vi "Test Log Critical Message.vi"(8 "error in (no error)":errorcluster, 11 "Test Case In":refnum<class "Logger Test.lvclass">) -> (0 "error out":errorcluster, 3 "Test Case Out":refnum<class "Logger Test.lvclass">)   [LabVIEW 2020, in "Logger Test.lvclass"]
uses:
  Logger Test.lvclass
  Logger Test.lvclass/Logger Test.ctl
  source/Framework Test Suite/Mock Log Handler/Mock Log Handler.lvclass
  source/Framework/Process/Process.lvclass
  source/Framework Test Suite/Mock Process/Mock Process.lvclass
  source/Framework/Logging/Logging.lvclass
  C:/Git/astemes-triarc-framework/source/Framework/Process/Process.lvclass
  C:/Git/astemes-triarc-framework/source/Framework/Base/Base.lvclass
  C:/Git/astemes-triarc-framework/source/Framework/Configuration File/Configuration File.lvclass
  C:/Git/astemes-triarc-framework/source/Framework/Configuration/Configuration.lvclass
  C:/Git/astemes-triarc-framework/source/Framework/Error Handler Interface/Error Handler Interface.lvclass
  C:/Git/astemes-triarc-framework/source/Framework/Logging/Logging.lvclass
  C:/Git/astemes-triarc-framework/source/Framework Test Suite/Mock Process/Mock Process.lvclass
  C:/Git/astemes-triarc-framework/source/Framework/Async Handler/Async Handler.lvclass
  C:/Git/astemes-triarc-framework/source/Framework/Helper Loop/Helper Loop.lvclass
  2651e2de-d45e-4850-8bc5-6c099aad78ff.vi
  C:/Git/astemes-triarc-framework/source/Framework Test Suite/Mock Log Handler/Mock Log Handler.lvclass
  5330ea77-6064-4515-90a2-c99ab62f2416.vi
  b0e1ba43-fbce-4c73-8e5c-724704fff6a6.vi
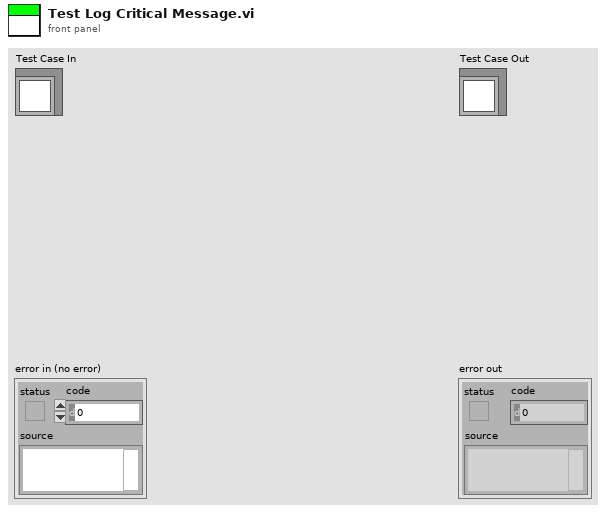
[diagram p1: front panel]
types:
  T1 = typedef "Mock Log Handler.lvclass/Log Entry.ctl" = cluster{"Level":string, "Source":string, "Message":string}
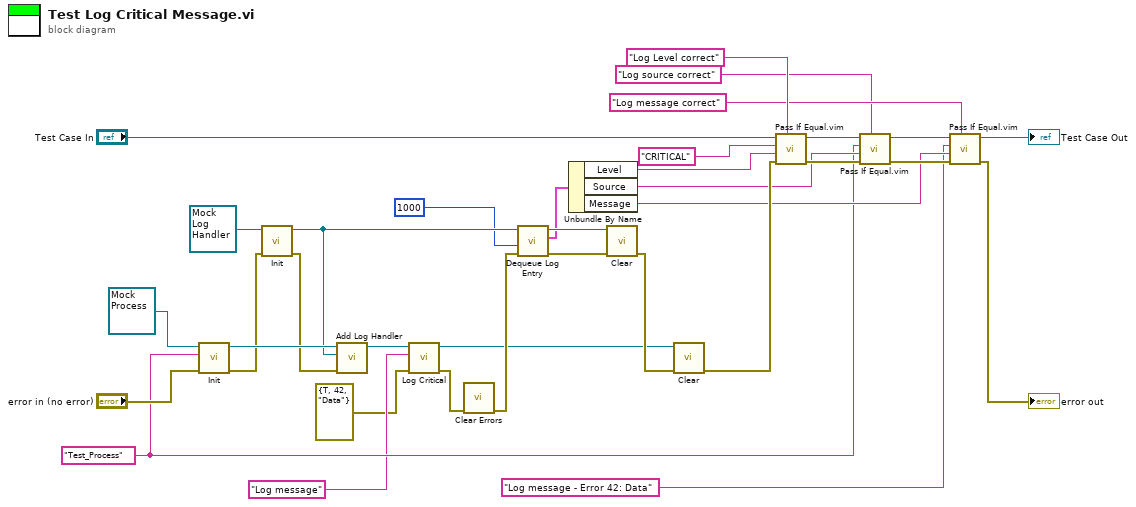
[diagram p0: block diagram]
diagram:
  w7 = "Test_Process" ("Name")
  n1 = call-dynamic "Init.vi"("error in (no error)"="error in (no error)", "Name"=w7, "Mock Process In"=refnum<class "Mock Process.lvclass"> refnum) -> ("error out"=w28:errorcluster, "Mock Process Out"=w32:refnum<class "Mock Process.lvclass">)  [unwired: 7 in]
  n2 = call-dynamic "Init.vi"("error in (no error)"=w28, "Mock Log Handler In"=refnum<class "Mock Log Handler.lvclass"> refnum ("Mock Log Handler.lvclass")) -> ("error out"=w27:errorcluster, "Mock Log Handler Out"=w24:refnum<class "Mock Log Handler.lvclass">)  [unwired: 8 in]
  n3 = call "Add Log Handler.vi"("error in (no error)"=w27, "Log Handler"=w24, "Process In"=w32) -> ("Process Out"=w22:refnum<class "Mock Process.lvclass">)  [unwired: 7 in, 1 out]
  n4 = call "Log Critical.vi"("error in (no error)"=errorcluster {"status"=TRUE, "code"=42, "source"="Data"}, "Message"="Log message", "Logging In"=w22) -> ("error out"=w4:errorcluster, "Logging Out"=w1:refnum<class "Mock Process.lvclass">)  [unwired: 7 in]
  n5 = call <vilib>:"Clear Errors.vi"("error in (no error)"=w4) -> ("error out"=w3:errorcluster)  [unwired: 5 in, 1 out]
  n6 = call "Dequeue Log Entry.vi"("error in (no error)"=w3, "timeout in ms (-1)"=1000, "Mock Log Handler in"=w24) -> ("error out"=w25:errorcluster, "Entry"=w20:T1, "Mock Log Handler out"=w26:refnum<class "Mock Log Handler.lvclass">)  [unwired: 5 in, 1 out]
  n7 = Unbundle By Name(w20) -> ("Level"=w19:string, "Source"=w9:string, "Message"=w8:string)
  n8 = call-dynamic "Clear.vi"("error in (no error)"=w25, "Mock Log Handler In"=w26) -> ("error out"=w21:errorcluster)  [unwired: 9 in]
  n9 = call-dynamic "Clear.vi"("error in (no error)"=w21, "Mock Process In"=w1) -> ("error out"=w13:errorcluster)  [unwired: 9 in]
  n10 = call "Pass If Equal.vim"("Description"="Log Level correct", "error in (no error)"=w13, "Actual"=w19, "Expected"="CRITICAL", "LUnit Test Case In"="Test Case In") -> ("error out"=w15:errorcluster, "LUnit Test Case Out"=w34:refnum<class "Logger Test.lvclass">)  [unwired: 5 in]
  n11 = call "Pass If Equal.vim"("Description"="Log source correct", "error in (no error)"=w15, "Actual"=w9, "Expected"=w7, "LUnit Test Case In"=w34) -> ("error out"=w14:errorcluster, "LUnit Test Case Out"=w17:refnum<class "Logger Test.lvclass">)  [unwired: 5 in]
  n12 = call "Pass If Equal.vim"("Description"="Log message correct", "error in (no error)"=w14, "Actual"=w8, "Expected"="Log message - Error 42: Data" ("Message"), "LUnit Test Case In"=w17) -> ("error out"=→"error out":errorcluster, "LUnit Test Case Out"=→"Test Case Out":refnum<class "Logger Test.lvclass">)  [unwired: 5 in]
